vi "CIC 滤波器设计.vi"() -> ()   [LabVIEW 2010]
uses:
  <vilib>/addons/Digital Filter Design/Multirate.llb/DFD MRate Filtering for Single Block (Wfm).vi
  <vilib>/measure/NI_MABase.lvlib
  <vilib>/addons/Digital Filter Design/NI_DigFilterLicensed.lvlib
panel:
  out "波形图":dbl[](graph)
  out "Y 2":dbl[](array[numeric])
  out "Y":dbl[](array[numeric])
  out "dt 2":dbl
  out "dt":dbl
  out "signal out 2":waveform(dbl)(graph) caption="信号输出"
  out "signal out":waveform(dbl)(graph) caption="信号输出"
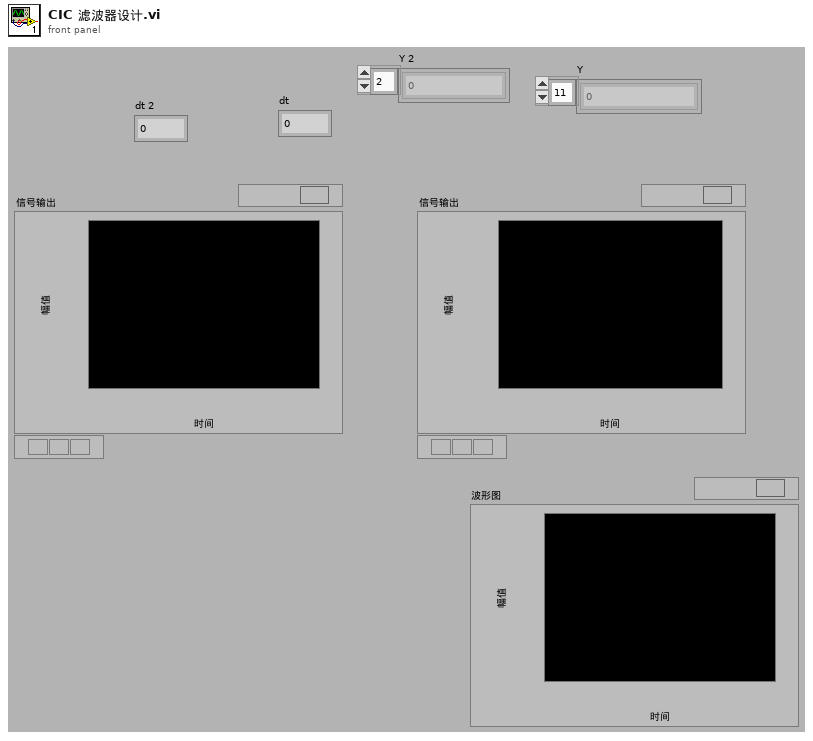
[diagram p1: front panel]
types:
  T1 = enum16{"Sine Wave", "Triangle Wave", "Square Wave", "Sawtooth Wave"}
  T2 = typedef "NI_DigFilterLicensed.lvlib/DFD Multirate Filter Obj.ctl" = cluster{"mMRate_Structure":enum16{"CIC", "FIR", "IIR", "Lattice"}, "mMRate_Mode":T3, "mMRate_Factor":i32, "mMRate_FIRParams":cluster{"mMRate_FIR_H":dbl[], "mMRate_FIR_IsNyquist?":bool, "mMRate_FIR_IsSymmetric?":bool}, "mMRate_CICParams":cluster{"mMRate_CIC_#Stage":i32, "mMRate_CIC_Lag":i32, "mMRate_CIC_Type":enum16{"Lowpass", "Highpass"}}, "mMRate_Order":i32, "mMRate_Version":string, "mMRate_Comments":string, "mMRate_RationalFactor":cluster{"mMRate_L":i32, "mMRate_M":i32}, "mMRate_Fs":dbl, "mMRate_Quantized?":bool, "mMRate_QFilterGain":dbl, "mMRate_CoefWl":i16, "mMRate_Scaling":cluster{"mMRate_ScaleByPowerOf2?":bool, "mMRate_ScaleType":T4}, "mMRate_InputWl":i16, "mMRate_OutputWl":i16, "mMRate_OutputMode":T5, "mMRate_MultMode":T6, "mMRate_BitPruning":bool, "mMRate_GainWl":i16, "mMRate_OutputFwl":i16, "mMRate_SumIwl":i16, "mMRate_InputIwl ":i16, "mMRate_SumWl":i16, "mMRate_CoefIwl":i16}
  T3 = typedef "NI_DigFilterLicensed.lvlib/DFD Multirate Mode.ctl" = i16
  T4 = typedef "NI_DigFilterLicensed.lvlib/DFD Coef Norm Type.ctl" = enum16{"No Norm", "Time Domain 1-Norm", "Time Domain 2-Norm", "Time Domain Inf-Norm"}
  T5 = typedef "NI_DigFilterLicensed.lvlib/DFD Round-off Mode.ctl" = enum16{"Nearest", "Truncation"}
  T6 = typedef "NI_DigFilterLicensed.lvlib/DFD FXP MRate Multiply Mode.ctl" = enum16{"Truncated", "Full"}
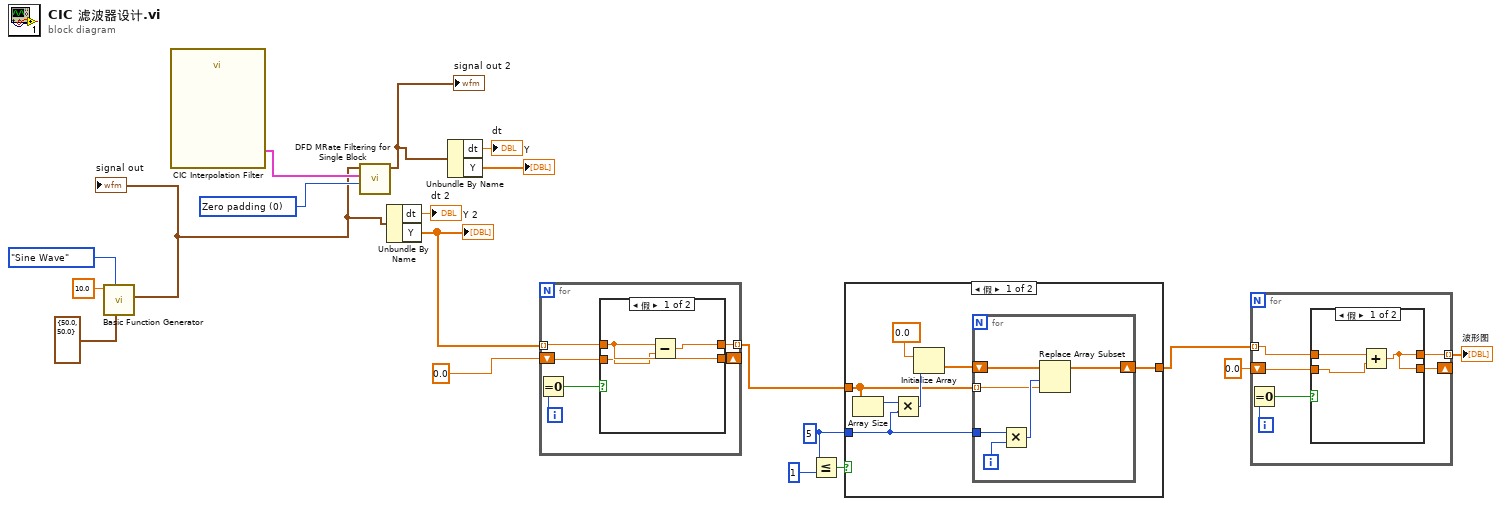
[diagram p0: block diagram]
diagram:
  w6 = 5 ("L")
  w15 = u16 0 items=["Zero padding", "Symmetric", "Periodic"] ("extension type")
  n1 = call <vilib>:"Basic Function Generator.vi"("sampling info"=cluster{"Fs":dbl, "#s":dbl} {"Fs"=50.0, "#s"=50.0}, "signal type"=T1."Sine Wave", "frequency"=10.0) -> ("signal out"=w11:waveform(dbl))  [unwired: 6 in, 2 out]
  "signal out" <- w11
  n2 = call "CIC Interpolation Filter"() -> ("CIC filter out"=w16:T2)  [unwired: 10 in, 1 out]
  n3 = call-poly <vilib>:"DFD MRate Filtering for Single Block.vi"("extension type"=w15, "multirate filter"=w16, "signal in"=w11) -> ("signal out"=w14:waveform(dbl))  [unwired: 7 in, 1 out]
  "signal out 2" <- w14
  n4 = Unbundle By Name(w11) -> ("dt"=→"dt 2":dbl, "Y"=w9:dbl[])
  "Y 2" <- w9
  n5 = Unbundle By Name(w14) -> ("dt"=→"dt":dbl, "Y"=→"Y":dbl[])
  n6 = for {
    tunnel: w9 -> [w24] mode=indexing
    tunnel: [w23] -> w4 mode=indexing
    shift-right: [w22] -> _
    shift-left: 0.0 -> [w21]
    i -> [w25]
    n7 = Equal To 0?(x=w25) -> (x = 0?=w20:bool)
    n8 = case shown="假" w20 {
      tunnel: w24 -> [w28 w29]
      tunnel: [w26 w29] -> w23
      tunnel: [w28 w29] -> w22
      tunnel: w21 -> [w27 _]
      frame False {
        n9 = Subtract(x=w28, y=w27) -> (x-y=w26:dbl)
      }
      frame True {
      }
    }
  }
  n10 = Less Or Equal?(x=w6, y=1) -> (x <= y?=w5:bool)
  n11 = case shown="假" w5 {
    tunnel: w4 -> [w33 w43]
    tunnel: w6 -> [w31 _]
    tunnel: [w30 w43] -> w3
    frame False {
      n12 = Array Size(array=w33) -> (size(s)=w32:i32)
      n13 = Multiply(x=w32, y=w31) -> (x*y=w35:i32)
      n14 = Initialize Array(0.0 ("Element Data"), w35) -> (w34:dbl[])
      n15 = for {
        shift-right: [w40] -> w30
        shift-left: w34 -> [w41]
        tunnel: w33 -> [w37] mode=indexing
        tunnel: w31 -> [w38]
        i -> [w42]
        n16 = Multiply(x=w38, y=w42) -> (x*y=w39:i32)
        n17 = Replace Array Subset(array=w41, new element=w37, index=w39) -> (w40:dbl[])
      }
    }
    frame True {
    }
  }
  n18 = for {
    tunnel: [w48] -> w1 mode=indexing
    shift-right: [w47] -> _
    shift-left: 0.0 ("Element Data") -> [w46]
    tunnel: w3 -> [w44] mode=indexing
    i -> [w49]
    n19 = Equal To 0?(x=w49) -> (x = 0?=w45:bool)
    n20 = case shown="假" w45 {
      tunnel: w44 -> [w52 w53]
      tunnel: [w50 w53] -> w48
      tunnel: [w50 w53] -> w47
      tunnel: w46 -> [w51 _]
      frame False {
        n21 = Add(x=w52, y=w51) -> (x+y=w50:dbl)
      }
      frame True {
      }
    }
  }
  "波形图" <- w1
